vi "Coor2Comm.vi"(1 "Numeric":dbl format="%#_13g", 2 "Cluster":T1 {"U" format="%#.5g"; "X" format="%#.5g"; "Y" format="%#.5g"; "Z" format="%#.5g"}) -> (0 "String":string)   [LabVIEW 2016]
uses:
  Control/Coordinate.ctl
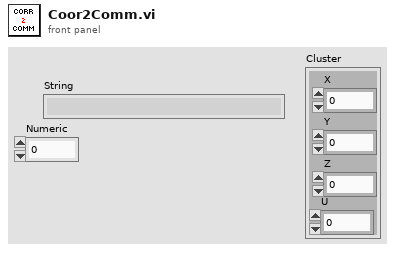
[diagram p1: front panel]
types:
  T1 = typedef "Coordinate.ctl" = cluster{"X":dbl, "Y":dbl, "Z":dbl, "U":dbl}
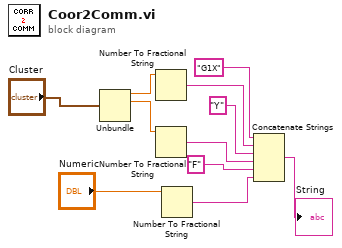
[diagram p0: block diagram]
diagram:
  n1 = Unbundle("Cluster") -> ("X"=w4:dbl, "Y"=w5:dbl)  [unwired: 2 out]
  n2 = Number To Fractional String(number=w4) -> (F-format string=w7:string)  [unwired: 3 in]
  n3 = Number To Fractional String(number=w5) -> (F-format string=w9:string)  [unwired: 3 in]
  n4 = Number To Fractional String(number="Numeric") -> (F-format string=w3:string)  [unwired: 3 in]
  n5 = Concatenate Strings("G1X", w7, "Y", w9, "F", w3) -> (→"String":string)
